vi "Get Timedloop Settings.vi"(8 "error in":errorcluster, 11 "Item Ref in":T2 format="%.0x") -> (0 "error out":errorcluster, 2 "Timed Loop Settings":T1={"Period(ms)"=2, "Priority"=100, "Processor"=-2}, 3 "Item Ref out":T2 format="%.0x")   [LabVIEW 2023, in "Vires VTD System Explorer.lvlib"]
uses:
  Vires VTD System Explorer.lvlib
  <vilib>/NI VeriStand/Custom Device API/Custom Device Item Ref.ctl
  Shared/Timedloop Settings.ctl
  Shared/Constants.vi
  <vilib>/NI VeriStand/Custom Device API/Get Item Property (Variant).vi
  Shared/Vires VTD Shared.lvlib
  <vilib>/NI VeriStand/Custom Device API/Custom Device API.lvlib
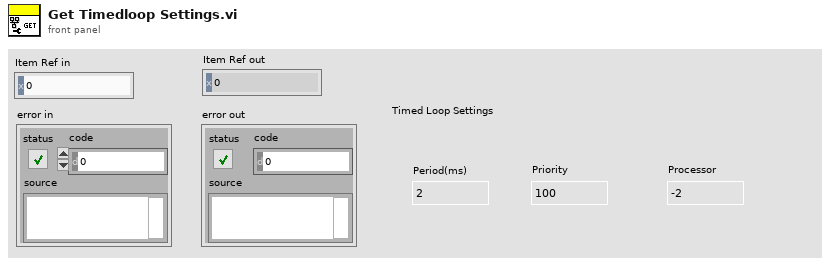
[diagram p1: front panel]
types:
  T1 = typedef "Vires VTD Shared.lvlib/Timedloop Settings.ctl" = cluster{"Period(ms)":i64, "Priority":i32, "Processor":i32}
  T2 = typedef "Custom Device API.lvlib/Custom Device Item Ref.ctl" = u64
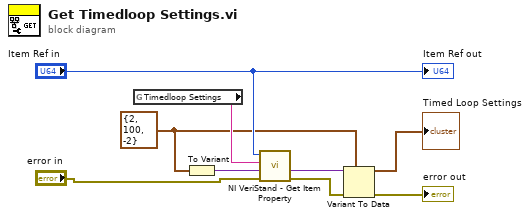
[diagram p0: block diagram]
diagram:
  w2 = T1 {"Period(ms)"=2, "Priority"=100, "Processor"=-2} ("Timed Loop Settings")
  n1 = global read "Constants.vi" "Timedloop Settings"() -> (w8:string)
  n2 = To Variant(anything=w2) -> (Variant=w7:variant)
  n3 = call-poly <vilib>:"NI VeriStand - Get Item Property.vi"("error in (no error)"="error in", "Default Value"=w7, "Property Name"=w8, "Item Ref in"="Item Ref in") -> ("error out"=w5:errorcluster, "Value"=w6:variant)  [unwired: 4 in, 2 out]
  n4 = Variant To Data(error in=w5, type=w2, Variant=w6) -> (data=→"Timed Loop Settings":T1, error out=→"error out":errorcluster)
  "Item Ref out" <- "Item Ref in"
